vi "Queue Lossy Insert.vi"(8 "error in (no error)":errorcluster, 9 "data":variant, 10 "event":string, 11 "queue name":string) -> (0 "error out":errorcluster, 2 "overflow?":bool, 3 "overflow element":T1)   [LabVIEW 2020]
uses:
  Control/Queue Data.ctl
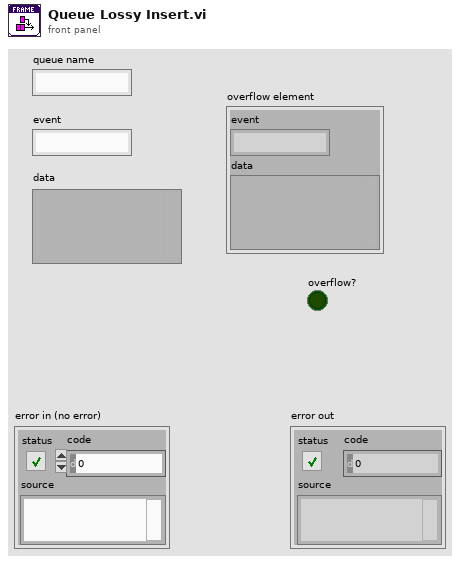
[diagram p1: front panel]
types:
  T1 = typedef "Queue Data.ctl" = cluster{"event":string, "data":variant}
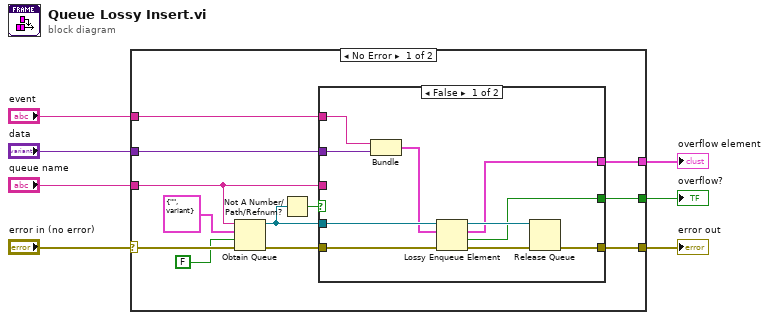
[diagram p0: block diagram]
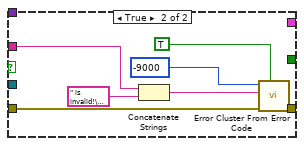
[diagram p2: hidden frame]
diagram:
  n1 = case shown="No Error" "error in (no error)" {
    selector: "error in (no error)" -> [w19 w37]
    tunnel: [w13 w37] -> w6
    tunnel: "queue name" -> [w14 _]
    tunnel: "event" -> [w11 _]
    tunnel: "data" -> [w10 _]
    tunnel: [w9 _] -> w2
    tunnel: [w8 _] -> w1
    frame No Error {
      n2 = Obtain Queue(name (unnamed)=w14, element data type=T1 {"event"="", "data"=variant} ("Cluster"), create if not found? (T)=FALSE, error in (no error)=w19) -> (queue out=w12:refnum<queue>, error out=w16:errorcluster)  [unwired: 1 in, 1 out]
      n3 = Not A Number/Path/Refnum?(number/path/refnum=w12) -> (NaN/Path/Refnum?=w15:bool)
      n4 = case shown="False" w15 {
        tunnel: w16 -> [w22 w32]
        tunnel: w14 -> [_ w31]
        tunnel: [w24 w30] -> w13
        tunnel: w12 -> [w29 _]
        tunnel: w11 -> [w27 _]
        tunnel: w10 -> [w28 _]
        tunnel: [w21 _] -> w9
        tunnel: [w20 _] -> w8
        frame False {
          n5 = Bundle("event"=w27, "data"=w28) -> (w26:cluster{"event":string, "data":variant})  [unwired: 1 in]
          n6 = Lossy Enqueue Element(queue=w29, element=w26, error in (no error)=w22) -> (queue out=w23:refnum<queue>, overflow element=w21:T1, overflow?=w20:bool, error out=w25:errorcluster)
          n7 = Release Queue(queue=w23, error in (no error)=w25) -> (error out=w24:errorcluster)  [unwired: 1 in, 2 out]
        }
        frame True {
          n8 = Concatenate Strings(w31, " is invalid!\nEnsure the queue has been created!" ("字符串")) -> (w34:string)
          n9 = call <vilib>:"Error Cluster From Error Code.vi"("show call chain? (False)"=TRUE, "error in (no error)"=w32, "error message (\"\")"=w34, "error code (0)"=-9000) -> ("error out"=w30:errorcluster)  [unwired: 5 in]
        }
      }
    }
    frame Error {
    }
  }
  "error out" <- w6
  "overflow element" <- w2
  "overflow?" <- w1
